vi "SetParam.vi"(7 "RS":bool, 8 "error in (no error)":errorcluster, 9 "Param to Set in":u16, 10 "Visa":refnum<visa-resource-name>, 11 "Filein":string) -> (0 "error out":errorcluster)   [LabVIEW 2017]
uses:
  <vilib>/Utility/miscctls.llb/LVMinMaxIncTypeDef.ctl
  <vilib>/Utility/config.llb/NI_LVConfig.lvlib
  <vilib>/Utility/config.llb/Read Key (String).vi
panel:
  out "RS Out":string
  out "Horizontal Progress Bar":i32(slide) min=0 max=50 scale=0.0..50.0
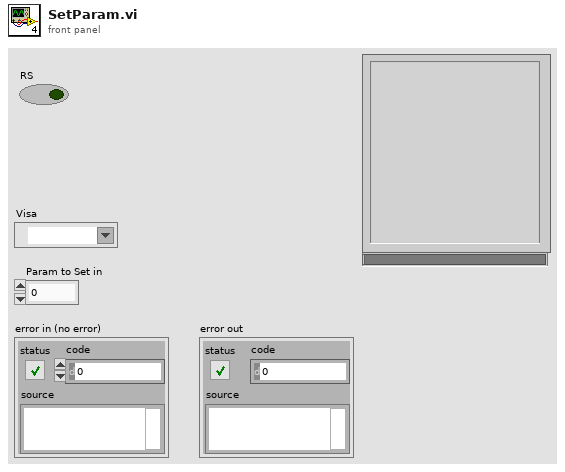
[diagram p1: front panel]
types:
  T1 = typedef "NI_LVConfig.lvlib/Config Data RefNum.ctl" = refnum<k1>
  T2 = typedef "LVMinMaxIncTypeDef.ctl" = cluster{"Minimum":dbl, "Maximum":dbl, "Increment":dbl}
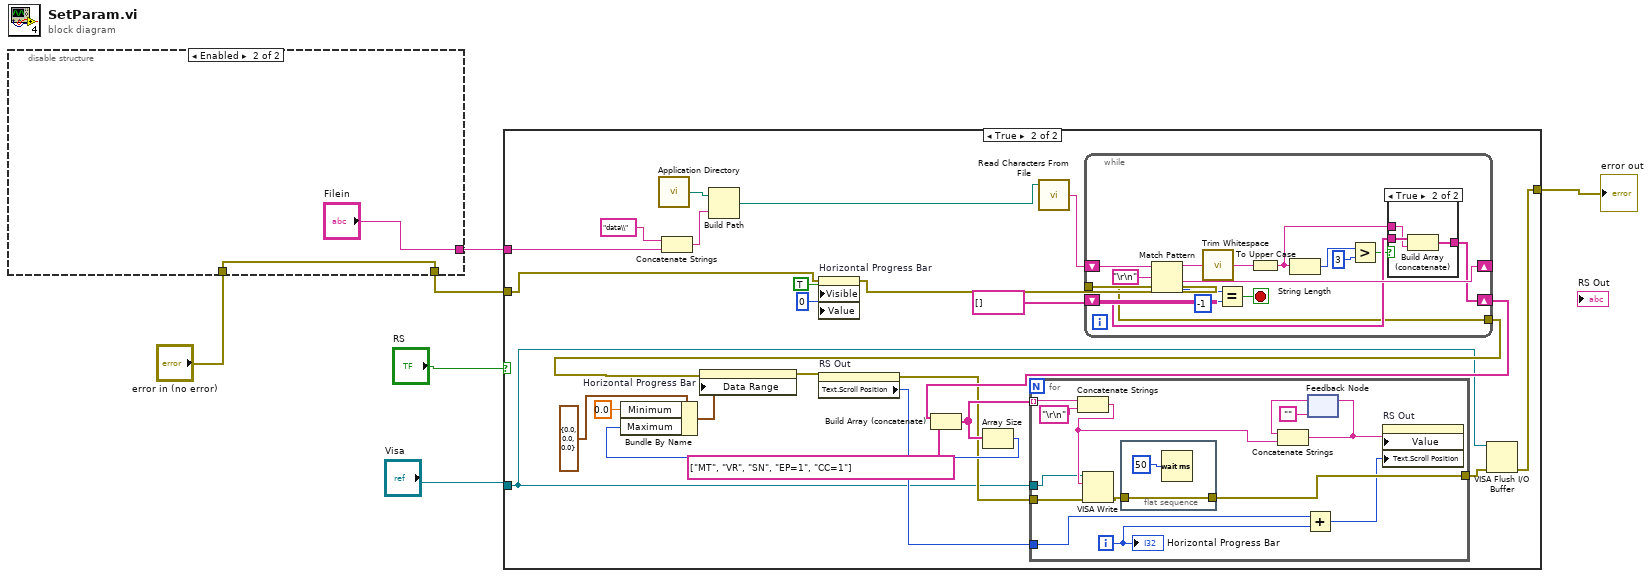
[diagram p0: block diagram]
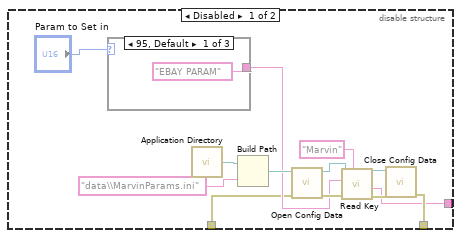
[diagram p2: hidden frame]
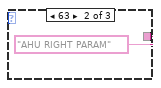
[diagram p3: hidden frame]
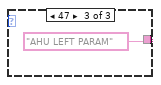
[diagram p4: hidden frame]
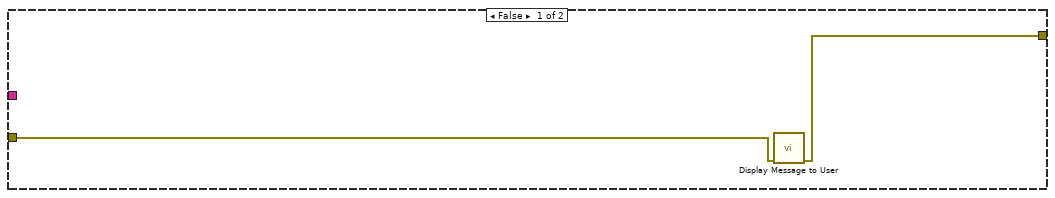
[diagram p5: hidden frame]
diagram:
  n1 = disable-structure shown="Enabled" {
    disable-tunnel: "error in (no error)" -> [w10 w24]
    disable-tunnel: [w9 w24] -> w2
    disable-tunnel: [w8 "Filein"] -> w1
    frame Disabled {
      n2 = case shown="95, Default" "Param to Set in" {
        tunnel: ["EBAY PARAM" ("section") "AHU RIGHT PARAM" ("section") "AHU LEFT PARAM" ("section")] -> w11
        frame 95, Default {
        }
        frame 63 {
        }
        frame 47 {
        }
      }
      n3 = call <vilib>:"Application Directory.vi"() -> ("Application Directory"=w19:path)
      n4 = Build Path(base path=w19, name or relative path="data\\MarvinParams.ini") -> (appended path=w15:path)
      n5 = call <vilib>:"Open Config Data.vi"("error in (no error)"=w10, "configuration file path"=w15) -> ("error out"=w14:errorcluster, "refnum"=w17:T1)  [unwired: 1 in, 7 out]
      n6 = call-poly <vilib>:"Read Key.vi"("section"="Marvin", "error in (no error)"=w14, "key"=w11, "refnum"=w17) -> ("error out"=w13:errorcluster, "value"=w8:string, "refnum out"=w12:T1)  [unwired: 2 in, 3 out]
      n7 = call <vilib>:"Close Config Data.vi"("error in (no error)"=w13, "refnum"=w12) -> ("error out"=w9:errorcluster)  [unwired: 8 in, 1 out]
    }
    frame Enabled {
    }
  }
  n8 = case shown="True" "RS" {
    tunnel: w2 -> [w26 w32]
    tunnel: [w25 w38] -> w5
    tunnel: "Visa" -> [_ w33]
    tunnel: w1 -> [_ w28]
    frame False {
      n9 = call "Display Message to User"("error in (no error)"=w26) -> ("error out"=w25:errorcluster)  [unwired: 9 in, 1 out]
    }
    frame True {
      n10 = call <vilib>:"Application Directory.vi"() -> ("Application Directory"=w30:path)
      n11 = Concatenate Strings("data\\" ("name or relative path"), w28) -> (w31:string)
      n12 = Build Path(base path=w30, name or relative path=w31) -> (appended path=w27:path)
      n13 = property on="Horizontal Progress Bar" class="Slide (strict)"(error in=w32, "Visible"=TRUE, "Value"=u8 0 ("Horizontal Progress Bar")) -> (error out=w40:errorcluster)  [unwired: 1 in, 1 out]
      n14 = call <vilib>:"Read Characters From File.vi"("file path (dialog if empty)"=w27) -> ("character string"=w50:string)  [unwired: 5 in, 3 out]
      n15 = while {
        shift-right: [w78] -> _
        shift-left: w50 -> [w79]
        shift-right: [w74] -> w41
        shift-left: string[] [] -> [w75]
        tunnel: w40 -> [w67]
        tunnel: [w67] -> w34
        stop <- w80 stop-if-true
        n16 = Match Pattern(string=w79, regular expression="\r\n") -> (before substring=w76:string, after substring=w78:string, offset past match=w77:i32)  [unwired: 1 in, 1 out]
        n17 = call <vilib>:"Trim Whitespace.vi"("string"=w76) -> ("trimmed string"=w73:string)  [unwired: 1 in]
        n18 = Equal?(x=w77, y=-1) -> (x = y?=w80:bool)
        n19 = To Upper Case(1:w73) -> (0:w71:string)
        n20 = String Length(string=w71) -> (length=w70:i32)
        n21 = Greater?(x=w70, y=3) -> (0:w68:bool)
        n22 = case shown="True" w68 {
          tunnel: w75 -> [w82 w85]
          tunnel: [w82 w84] -> w74
          tunnel: w71 -> [_ w83]
          frame False {
          }
          frame True {
            n23 = Build Array (concatenate)(w85, w83) -> (w84:string[])
          }
        }
      }
      n24 = Build Array (concatenate)(w41, string[] ["MT", "VR", "SN", "EP=1", "CC=1"] ("array")) -> (w46:string[])
      n25 = Array Size(array=w46) -> (size(s)=w42:i32)
      n26 = Bundle By Name(cluster=T2 {"Minimum"=0.0, "Maximum"=0.0, "Increment"=0.0} ("Data Entry Limits"), "Minimum"=0.0, "Maximum"=w42) -> (w44:T2)
      n27 = property on="Horizontal Progress Bar" class="Slide (strict)"(error in=w34, "Data Range"=w44) -> (error out=w37:errorcluster)  [unwired: 1 in, 1 out]
      n28 = property on="RS Out" class="Str"(error in=w37) -> (error out=w36:errorcluster, "Text.Scroll Position"=w35:u32)  [unwired: 1 in, 1 out]
      n29 = for {
        tunnel: w46 -> [w59] mode=indexing
        tunnel: w36 -> [w64]
        tunnel: [w56] -> w39
        tunnel: w35 -> [w55]
        tunnel: w33 -> [w52]
        i -> [w54]
        n30 = Concatenate Strings(w59, "\r\n" ("string")) -> (w57:string)
        n31 = VISA Write(VISA resource name=w52, write buffer=w57, error in (no error)=w64) -> (error out=w63:errorcluster)  [unwired: 2 out]
        n32 = flat-sequence {
          tunnel: w63 -> [w65]
          tunnel: [w65] -> w56
          frame #0 {
            n33 = Wait (ms)(milliseconds to wait=u32 50) -> ()  [unwired: 1 out]
          }
        }
        n34 = Add(x=w55, y=w54) -> (x+y=w53:u32)
        n35 = feedback #1("") -> (w61:string)
        n36 = Concatenate Strings(w61, w57) -> (w62:string)
        n37 = feedback-in #1(w62) -> ()
        n38 = property on="RS Out" class="Str"("Value"=w62, "Text.Scroll Position"=w53) -> ()  [unwired: 2 in, 2 out]
        "Horizontal Progress Bar" <- w54
      }
      n39 = VISA Flush I/O Buffer(VISA resource name=w33, error in (no error)=w39) -> (error out=w38:errorcluster)  [unwired: 1 in, 1 out]
    }
  }
  "error out" <- w5
